vi "PathPlanner_TrajectoryState_Reverse.vi"(11 "PathPlannerState":T1={"TimeSeconds"=0.0, "VelocityMPS"=0.0, "AccerationMpsSq"=0.0, "HeadingAngularVelRadPerSec"=0.0, "PositionMeters"={"X"=0.0, "Y"=1.0}, "Heading"={"VALUE"=0.0, "COS"=1.0, "SIN"=0.0}, "TargetHolonomicRotation"={"VALUE"=0.0, "COS"=1.0, "SIN"=0.0}, "CurvatureRadPerMeter"=0.0, "PathPlannerConstraints"={"MaxVelocityMps;"=0.0, "MaxAccelerationMpsSq;"=0.0, "MaxAngularVelRadPsEc;"=0.0, "MaxAngularAccRadPSecSq"=0.0, "Exists"=FALSE}, "DeltaPos"=0.0} {"TargetHolonomicRotation"."SIN" format="%13.4f"; "TargetHolonomicRotation"."COS" format="%13.4f"; "TargetHolonomicRotation"."VALUE" format="%13.4f"; "Heading"."SIN" format="%13.4f"; "Heading"."COS" format="%13.4f"; "Heading"."VALUE" format="%13.4f"; "PositionMeters"."Y" format="%14.3f"; "PositionMeters"."X" format="%14.3f"}) -> (3 "Reversed State":T1={"TimeSeconds"=0.0, "VelocityMPS"=0.0, "AccerationMpsSq"=0.0, "HeadingAngularVelRadPerSec"=0.0, "PositionMeters"={"X"=0.0, "Y"=0.0}, "Heading"={"VALUE"=0.0, "COS"=1.0, "SIN"=0.0}, "TargetHolonomicRotation"={"VALUE"=0.0, "COS"=1.0, "SIN"=0.0}, "CurvatureRadPerMeter"=0.0, "PathPlannerConstraints"={"MaxVelocityMps;"=0.0, "MaxAccelerationMpsSq;"=0.0, "MaxAngularVelRadPsEc;"=0.0, "MaxAngularAccRadPSecSq"=0.0, "Exists"=FALSE}, "DeltaPos"=0.0} {"TargetHolonomicRotation"."SIN" format="%13.4f"; "TargetHolonomicRotation"."COS" format="%13.4f"; "TargetHolonomicRotation"."VALUE" format="%13.4f"; "Heading"."SIN" format="%13.4f"; "Heading"."COS" format="%13.4f"; "Heading"."VALUE" format="%13.4f"; "PositionMeters"."Y" format="%14.3f"; "PositionMeters"."X" format="%14.3f"})   [LabVIEW 2019, in "PathPlanner.lvlib"]
doc: "Get the state reversed, used for following a trajectory reversed with a differential drivetrain\n \nInputs: \n - trajectoryState - cluster - this trajectory state\n\nOutputs:\n - ReversedState- trajectorystate - The reversed state"
uses:
  PathPlanner.lvlib
  TypeDef/PathPlannerTrajectoryState.ctl
  <vilib>/Rock Robotics/WPI/ThirdParty/JAS_Junk/TrajLib/TypeDef/TRANSLATION2D.ctl
  <vilib>/Rock Robotics/WPI/ThirdParty/JAS_Junk/TrajLib/TypeDef/ROTATION2D.ctl
  TypeDef/PathPlannerPathConstraints.ctl
  <vilib>/Rock Robotics/WPI/ThirdParty/JAS_Junk/TrajLib/Rotation2d_GetRadians.vi
  <vilib>/Rock Robotics/WPI/ThirdParty/JAS_Junk/TrajLib/Conv_Radians_Deg.vi
  <vilib>/Rock Robotics/WPI/ThirdParty/JAS_Junk/TrajLib/Conv_Deg_Radians.vi
  <vilib>/Rock Robotics/WPI/ThirdParty/JAS_Junk/TrajLib/Rotation2d_CreateAngle.vi
  <vilib>/Rock Robotics/WPI/ThirdParty/JAS_Junk/TrajLib/Trajectory_Library.lvlib
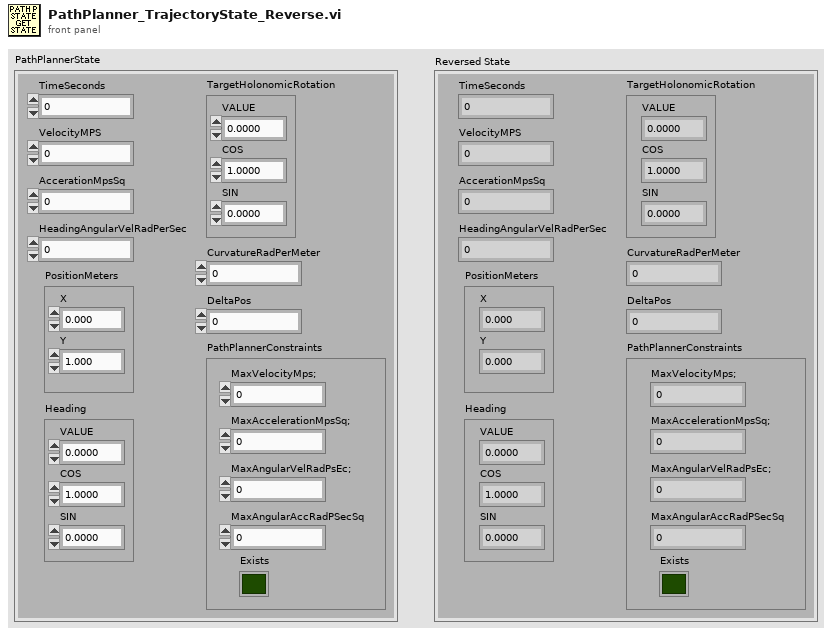
[diagram p1: front panel]
types:
  T1 = typedef "PathPlanner.lvlib/PathPlannerTrajectoryState.ctl" = cluster{"TimeSeconds":dbl, "VelocityMPS":dbl, "AccerationMpsSq":dbl, "HeadingAngularVelRadPerSec":dbl, "PositionMeters":T2, "Heading":T3, "TargetHolonomicRotation":T3, "CurvatureRadPerMeter":dbl, "PathPlannerConstraints":T4, "DeltaPos":dbl}
  T2 = typedef "Trajectory_Library.lvlib/TRANSLATION2D.ctl" = cluster{"X":dbl, "Y":dbl}
  T3 = typedef "Trajectory_Library.lvlib/ROTATION2D.ctl" = cluster{"VALUE":dbl, "COS":dbl, "SIN":dbl}
  T4 = typedef "PathPlanner.lvlib/PathPlannerPathConstraints.ctl" = cluster{"MaxVelocityMps;":dbl, "MaxAccelerationMpsSq;":dbl, "MaxAngularVelRadPsEc;":dbl, "MaxAngularAccRadPSecSq":dbl, "Exists":bool}
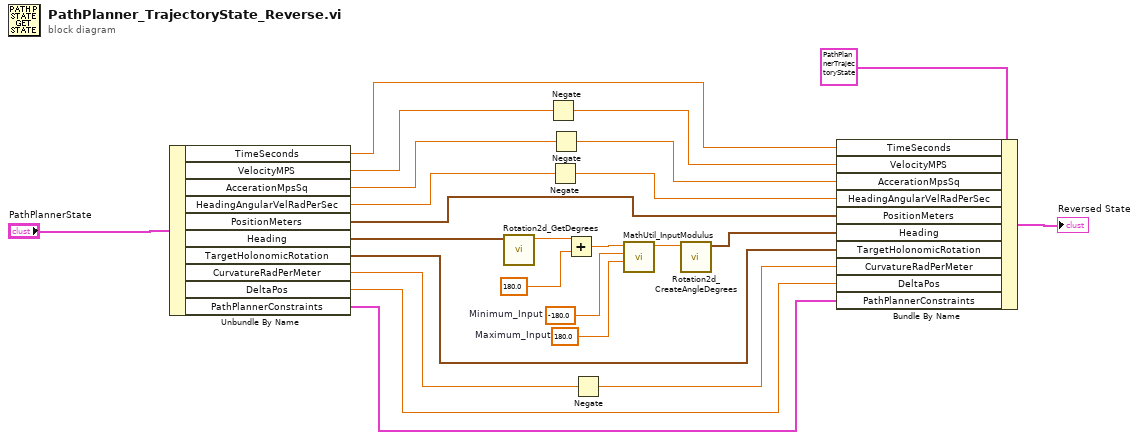
[diagram p0: block diagram]
diagram:
  w10 = -180.0  # Minimum_Input
  w9 = 180.0  # Maximum_Input
  n1 = Unbundle By Name("PathPlannerState") -> ("TimeSeconds"=w21:dbl, "VelocityMPS"=w20:dbl, "AccerationMpsSq"=w19:dbl, "HeadingAngularVelRadPerSec"=w18:dbl, "PositionMeters"=w14:T2, "Heading"=w13:T3, "TargetHolonomicRotation"=w5:T3, "CurvatureRadPerMeter"=w4:dbl, "DeltaPos"=w2:dbl, "PathPlannerConstraints"=w1:T4)
  n2 = call <vilib>:"Rotation2d_GetDegrees.vi"("in ROTATION"=w13) -> ("AngleDegrees"=w12:dbl)  [unwired: 10 in]
  n3 = Negate(x=w20) -> (-x=w17:dbl)
  n4 = Negate(x=w18) -> (-x=w15:dbl)
  n5 = Negate(x=w19) -> (-x=w16:dbl)
  n6 = Add(x=w12, y=180.0) -> (x+y=w8:dbl)
  n7 = Negate(x=w4) -> (-x=w3:dbl)
  n8 = call <vilib>:"MathUtil_InputModulus.vi"("Maximum_Input"=w9, "Minimum_Input"=w10, "Input"=w8) -> ("modulus"=w7:dbl)  [unwired: 8 in]
  n9 = call <vilib>:"Rotation2d_CreateAngleDegrees.vi"("Angle_Degrees"=w7) -> ("ROTATION"=w6:T3)  [unwired: 10 in]
  n10 = Bundle By Name(cluster=T1 {"TimeSeconds"=0.0, "VelocityMPS"=0.0, "AccerationMpsSq"=0.0, "HeadingAngularVelRadPerSec"=0.0, "PositionMeters"={"X"=0.0, "Y"=0.0}, "Heading"={"VALUE"=0.0, "COS"=1.0, "SIN"=0.0}, "TargetHolonomicRotation"={"VALUE"=0.0, "COS"=1.0, "SIN"=0.0}, "CurvatureRadPerMeter"=0.0, "PathPlannerConstraints"={"MaxVelocityMps;"=0.0, "MaxAccelerationMpsSq;"=0.0, "MaxAngularVelRadPsEc;"=0.0, "MaxAngularAccRadPSecSq"=0.0, "Exists"=FALSE}, "DeltaPos"=0.0} ("PathPlannerState"), "TimeSeconds"=w21, "VelocityMPS"=w17, "AccerationMpsSq"=w16, "HeadingAngularVelRadPerSec"=w15, "PositionMeters"=w14, "Heading"=w6, "TargetHolonomicRotation"=w5, "CurvatureRadPerMeter"=w3, "DeltaPos"=w2, "PathPlannerConstraints"=w1) -> (→"Reversed State":T1)
